vi "Mapping Countdown Simulation.vi"() -> ()   [LabVIEW 2010]
uses:
  TypeDefs/Mapping Drive Params.ctl
  ESA-C/TypeDefs/ESA-C Set Positions.ctl
  TypeDefs/Mapping Spectra Params.ctl
panel:
  out "X-Time (s)":dbl
  out "Total Time (s)":dbl
  out "Progress":i16
  in  "Messung starten":bool=TRUE
  out "Schieberegler":dbl(slide) scale=0.0..100.0
  out "Time String":string
  in  "Drive Velocity":dbl=5.0 caption="Velocity (V/s)" min=10.0 max=160.0 step=0.1 format="%.1f"
  in  "Mapping Spectra Settings":T1={"Integration Time"=10.0, "Repetitions"=10, "Mapping Spectra"=FALSE} {"Repetitions" min=1 max=100 step=1; "Integration Time" min=0.5 max=6000.0 step=1.0 format="%.1f"}
  in  "Drive New Abs. Positions":T2 {"Drive X Set" min=10.0 max=160.0 step=0.1 format="%.1f"; "Drive Z Set" min=10.0 max=160.0 step=0.1 format="%.1f"; "Drive Y Set" min=10.0 max=160.0 step=0.1 format="%.1f"}
  in  "Mapping Drive Parameters":T3={"X Start Position"=0.0, "X Stop Position"=10.0, "Y Start Position"=0.0, "Y Stop Position"=10.0, "Step Size"=2.0} {"Step Size" min=0.1 max=30.0 step=0.1 format="%.1f"; "Y Stop Position" min=0.0 max=30.0 step=0.1 format="%.1f"; "Y Start Position" min=0.0 max=30.0 step=0.1 format="%.1f"; "X Stop Position" min=0.0 max=30.0 step=0.1 format="%.1f"; "X Start Position" min=0.0 max=30.0 step=0.1 format="%.1f"}
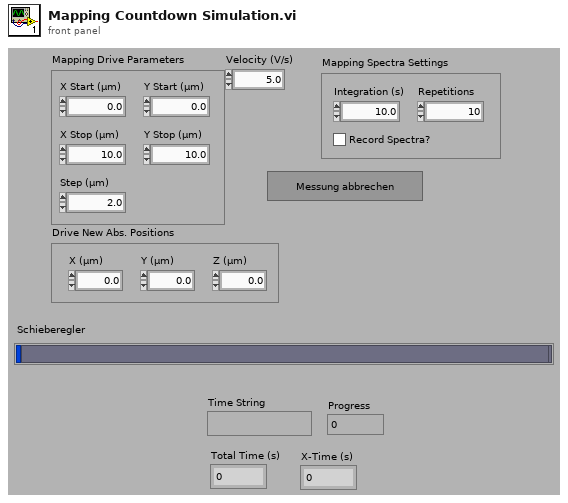
[diagram p1: front panel]
types:
  T1 = typedef "Mapping Spectra Params.ctl" = cluster{"Integration Time":dbl, "Repetitions":u16, "Mapping Spectra":bool}
  T2 = typedef "ESA-C Set Positions.ctl" = cluster{"Drive X Set":dbl, "Drive Y Set":dbl, "Drive Z Set":dbl}
  T3 = typedef "Mapping Drive Params.ctl" = cluster{"X Start Position":dbl, "X Stop Position":dbl, "Y Start Position":dbl, "Y Stop Position":dbl, "Step Size":dbl}
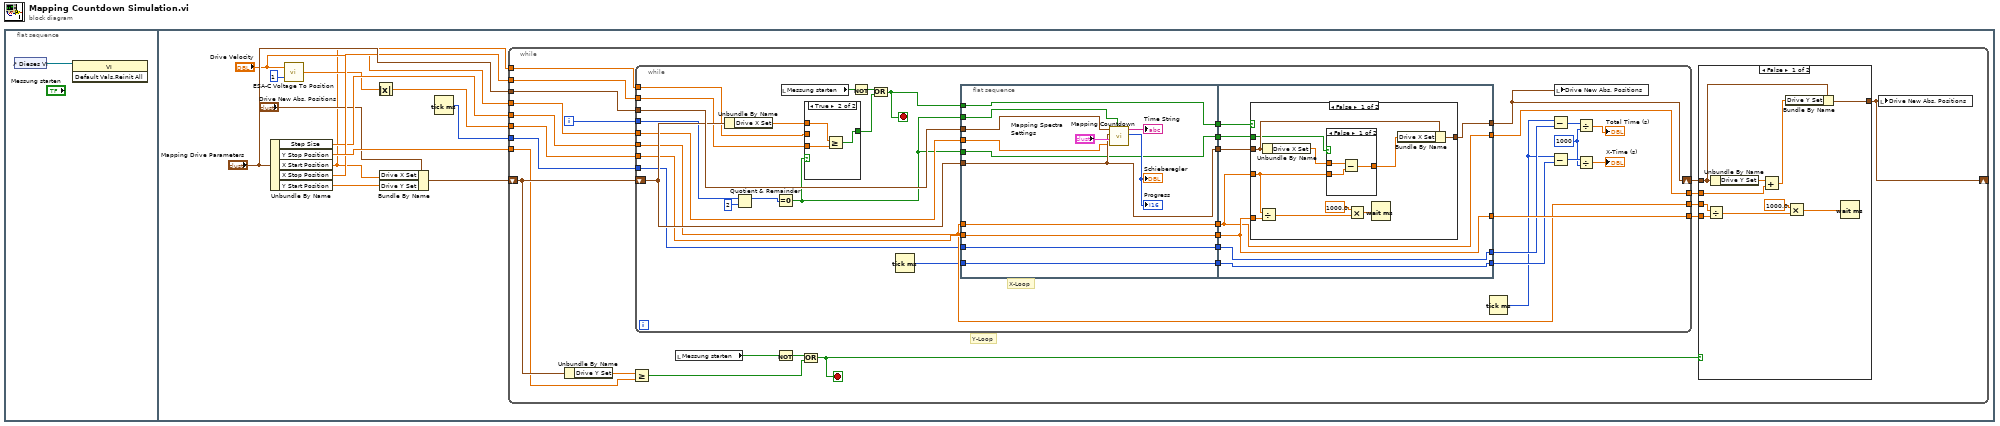
[diagram p0: block diagram]
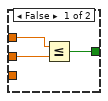
[diagram p3: hidden frame]
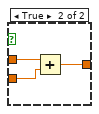
[diagram p4: hidden frame]
diagram:
  n1 = flat-sequence {
    frame #0 {
      n2 = control-ref of="Dieses VI"() -> (w1:refnum<vi>)
      n3 = invoke class="VI" method="Default Vals.Reinit All"(reference=w1) -> ()  [unwired: 2 in, 3 out]
    }
    frame #1 {
      n4 = Unbundle By Name("Mapping Drive Parameters") -> ("Step Size"=w10:dbl, "Y Stop Position"=w13:dbl, "X Start Position"=w5:dbl, "X Stop Position"=w12:dbl, "Y Start Position"=w4:dbl)
      n5 = call "ESA-C Voltage To Position.vi"("Axis"=1, "Voltage (V)"="Drive Velocity") -> ("Position (µm)"=w8:dbl)
      n6 = Absolute Value(x=w8) -> (abs(x)=w7:dbl)
      n7 = Bundle By Name(cluster="Drive New Abs. Positions", "Drive X Set"=w5, "Drive Y Set"=w4) -> (w3:T2)
      n8 = Tick Count (ms)() -> (millisecond timer value=w2:u32)
      n9 = while {
        shift-right: [w17] -> _
        shift-left: w3 -> [w29]
        tunnel: "Mapping Drive Parameters" -> [w30]
        tunnel: w13 -> [w28]
        tunnel: w5 -> [w27]
        tunnel: w12 -> [w26]
        tunnel: "Drive Velocity" -> [w25]
        tunnel: w10 -> [w24]
        tunnel: w7 -> [w23]
        tunnel: w2 -> [w15]
        i -> [w22]
        stop <- w19 stop-if-true
        # "Y-Loop"
        n10 = Unbundle By Name(w29) -> ("Drive Y Set"=w34:dbl)
        n11 = Greater Or Equal?(x=w34, y=w28) -> (x >= y?=w31:bool)
        n12 = while {
          shift-right: [w59] -> w18
          shift-left: w29 -> [w74]
          tunnel: w30 -> [w80]
          tunnel: w27 -> [w73]
          tunnel: w26 -> [w72]
          tunnel: w25 -> [w71]
          tunnel: w24 -> [w66]
          tunnel: w23 -> [w68]
          tunnel: w22 -> [w70]
          tunnel: [w66] -> w21
          tunnel: [w69] -> w20
          tunnel: [w58] -> w16
          tunnel: w15 -> [w56]
          stop <- w64 stop-if-true
          w47 = u32 1000 ("y")
          # "X-Loop"
          n13 = Unbundle By Name(w74) -> ("Drive X Set"=w75:dbl)
          n14 = Quotient & Remainder(x=w70, y=2) -> (x-y*floor(x/y)=w77:i32)  [unwired: 1 out]
          n15 = Equal To 0?(x=w77) -> (x = 0?=w60:bool)
          n16 = local read "Messung starten"() -> (w79:bool)
          n17 = case shown="True" w60 {
            tunnel: w75 -> [w82 w85]
            tunnel: w72 -> [_ w87]
            tunnel: [w84 w86] -> w62
            tunnel: w73 -> [w83 _]
            frame False {
              n18 = Less Or Equal?(x=w82, y=w83) -> (x <= y?=w84:bool)
            }
            frame True {
              n19 = Greater Or Equal?(x=w85, y=w87) -> (x >= y?=w86:bool)
            }
          }
          n20 = Not(x=w79) -> (.not. x?=w78:bool)
          n21 = Or(x=w78, y=w62) -> (x .or. y?=w64:bool)
          n22 = Tick Count (ms)() -> (millisecond timer value=w51:u32)
          n23 = flat-sequence {
            tunnel: w74 -> [w97]
            tunnel: [w97] -> w81
            tunnel: w80 -> [w96]
            tunnel: w60 -> [w95]
            tunnel: w71 -> [w94]
            tunnel: w68 -> [w93]
            tunnel: [w93] -> w67
            tunnel: w66 -> [w92]
            tunnel: [w92] -> w65
            tunnel: w64 -> [w91]
            tunnel: [w91] -> w63
            tunnel: [w90] -> w61
            tunnel: w60 -> [w90]
            tunnel: [w89] -> w57
            tunnel: w56 -> [w89]
            tunnel: [w88] -> w52
            tunnel: w51 -> [w88]
            tunnel: w81 -> [w106]
            tunnel: [w105] -> w59
            tunnel: [w108] -> w69
            tunnel: w67 -> [w108]
            tunnel: w65 -> [w103]
            tunnel: w63 -> [w107]
            tunnel: w61 -> [w104]
            tunnel: [w103] -> w58
            tunnel: [w102] -> w55
            tunnel: w57 -> [w102]
            tunnel: [w101] -> w50
            tunnel: w52 -> [w101]
            frame #0 {
              n24 = call "Mapping Countdown.vi"("Forward?"=w95, "Drive Velocity"=w94, "Mapping Spectra Settings"="Mapping Spectra Settings", "Drive New Abs. Positions"=w97, "Mapping Drive Parameters"=w96) -> ("Progress"=→"Schieberegler" →"Progress":i16, "Time String"=→"Time String":string)  [unwired: 5 in]
            }
            frame #1 {
              n25 = case shown="False" w107 {
                tunnel: w103 -> [w110 _]
                tunnel: w108 -> [w116 _]
                tunnel: w106 -> [w111 w125]
                tunnel: [w112 w125] -> w105
                tunnel: w104 -> [w109 _]
                frame False {
                  n26 = Divide(x=w110, y=w116) -> (x/y=w115:dbl)
                  n27 = Unbundle By Name(w111) -> ("Drive X Set"=w114:dbl)
                  n28 = case shown="False" w109 {
                    tunnel: w114 -> [w120 w124]
                    tunnel: [w121 w123] -> w113
                    tunnel: w110 -> [w119 w122]
                    frame False {
                      n29 = Subtract(x=w120, y=w119) -> (x-y=w121:dbl)
                    }
                    frame True {
                      n30 = Add(x=w124, y=w122) -> (x+y=w123:dbl)
                    }
                  }
                  n31 = Multiply(x=1000.0, y=w115) -> (x*y=w117:dbl)
                  n32 = Wait (ms)(milliseconds to wait=w117) -> ()  [unwired: 1 out]
                  n33 = Bundle By Name(cluster=w111, "Drive X Set"=w113) -> (w112:T2)
                }
                frame True {
                }
              }
            }
          }
          n34 = Tick Count (ms)() -> (millisecond timer value=w49:u32)
          n35 = Subtract(x=w49, y=w55) -> (x-y=w54:u32)
          n36 = Subtract(x=w49, y=w50) -> (x-y=w48:u32)
          n37 = local write "Drive New Abs. Positions"(w59) -> ()
          n38 = Divide(x=w54, y=w47) -> (x/y=→"Total Time (s)":dbl)
          n39 = Divide(x=w48, y=w47) -> (x/y=→"X-Time (s)":dbl)
        }
        n40 = local read "Messung starten"() -> (w32:bool)
        n41 = Not(x=w32) -> (.not. x?=w33:bool)
        n42 = Or(x=w33, y=w31) -> (x .or. y?=w19:bool)
        n43 = case shown="False" w19 {
          tunnel: w20 -> [w42 _]
          tunnel: w21 -> [w40 _]
          tunnel: w18 -> [w37 w45]
          tunnel: [w36 w45] -> w17
          tunnel: w16 -> [w35 _]
          frame False {
            n44 = Divide(x=w40, y=w42) -> (x/y=w41:dbl)
            n45 = Unbundle By Name(w37) -> ("Drive Y Set"=w39:dbl)
            n46 = Add(x=w39, y=w35) -> (x+y=w38:dbl)
            n47 = Bundle By Name(cluster=w37, "Drive Y Set"=w38) -> (w36:T2)
            n48 = Multiply(x=1000.0, y=w41) -> (x*y=w43:dbl)
            n49 = Wait (ms)(milliseconds to wait=w43) -> ()  [unwired: 1 out]
          }
          frame True {
          }
        }
        n50 = local write "Drive New Abs. Positions"(w17) -> ()
      }
    }
  }
